vi "Map To Bitmask.vi"(8 "error in (no error)":errorcluster, 10 "64-bitmask Input":u64, 11 "ElectrodeGrid in":refnum<class "ElectrodeGrid.lvclass">) -> (0 "error out":errorcluster, 2 "64-bitmask Output":u64, 3 "ElectrodeGrid out":refnum<class "ElectrodeGrid.lvclass">)   [LabVIEW 2017, in "ElectrodeGrid.lvclass"]
doc: "This VI will map the electrode grid array to ON-OFF bits in the 64 bit data buffer.\n\nThe electrode boolean array and bitmask map come from the object's properties."
uses:
  ElectrodeGrid.lvclass
  ElectrodeGrid.lvclass/ElectrodeGrid.ctl
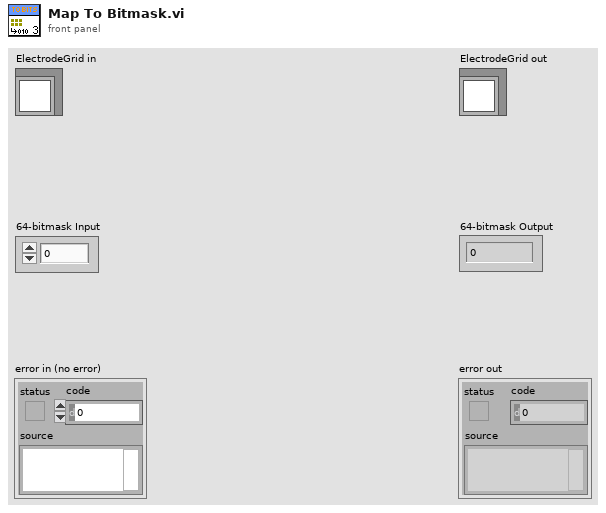
[diagram p1: front panel]
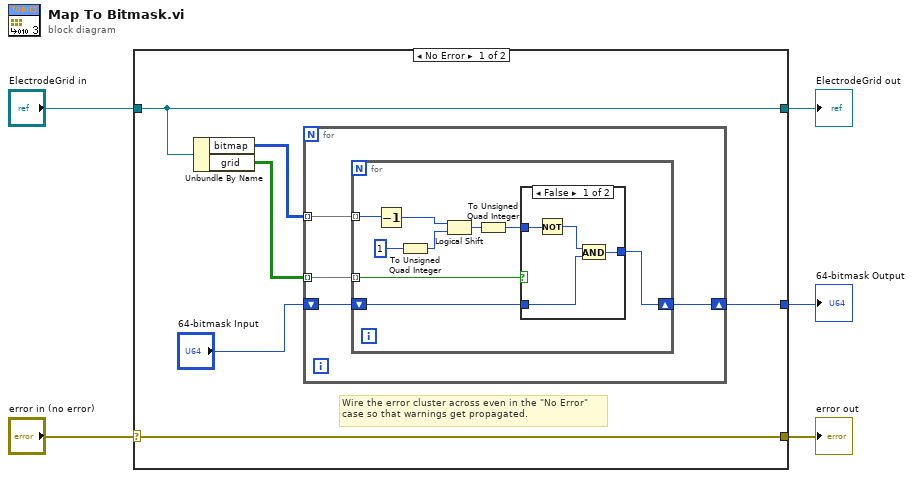
[diagram p0: block diagram]
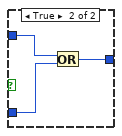
[diagram p2: hidden frame]
diagram:
  n1 = case shown="No Error" "error in (no error)" {
    selector: "error in (no error)" -> [w11 w33]
    tunnel: [w11 w33] -> w4
    tunnel: [w10 w32] -> w2
    tunnel: "ElectrodeGrid in" -> [w10 w32]
    tunnel: [w7 _] -> w1
    frame No Error {
      # "Wire the error cluster across even in the \"No Error\"\ncase so that warnings get propagated."
      n2 = Unbundle By Name(w10) -> ("bitmap"=w8:u8[][], "grid"=w9:bool[][])
      n3 = for {
        tunnel: w9 -> [w14] mode=indexing
        tunnel: w8 -> [w15] mode=indexing
        shift-right: [w12] -> w7
        shift-left: "64-bitmask Input" -> [w13]
        n4 = for {
          tunnel: w15 -> [w24] mode=indexing
          tunnel: w14 -> [w18] mode=indexing
          shift-right: [w16] -> w12
          shift-left: w13 -> [w17]
          n5 = Decrement(x=w24) -> (x-1=w21:u8)
          n6 = To Unsigned Quad Integer(1:u64 1 ("number")) -> (0:w22:u64)
          n7 = Logical Shift(y=w21, x=w22) -> (x << y=w23:u64)
          n8 = To Unsigned Quad Integer(1:w23) -> (0:w20:u64)
          n9 = case shown="False" w18 {
            tunnel: w20 -> [w28 w31]
            tunnel: w17 -> [w26 w30]
            tunnel: [w25 w29] -> w16
            frame False {
              n10 = Not(x=w28) -> (.not. x?=w27:u64)
              n11 = And(x=w27, y=w26) -> (x .and. y?=w25:u64)
            }
            frame True {
              n12 = Or(x=w31, y=w30) -> (x .or. y?=w29:u64)
            }
          }
        }
      }
    }
    frame Error {
    }
  }
  "error out" <- w4
  "ElectrodeGrid out" <- w2
  "64-bitmask Output" <- w1
